vi "AWG Set Gain & Offset.vi"(6 "Pins":string[](array[string]), 8 "error in":errorcluster, 9 "Offset":dbl=0.5, 10 "Gain":dbl=0.5, 11 "Semiconductor Module Context In":T1) -> (0 "error out":errorcluster, 2 "Instruments Handle Out":refnum<k15>[](array[refnum]), 3 "Semiconductor Module Context Out":T1)   [LabVIEW 2013]
uses:
  <vilib>/NI_TestStand_SemiconductorModule/NI_TestStand_Semiconductor_Module.lvlibp/PinMap/General/SemiconductorModuleContext.ctl
  <vilib>/NI_TestStand_SemiconductorModule/NI_TestStand_Semiconductor_Module.lvlibp
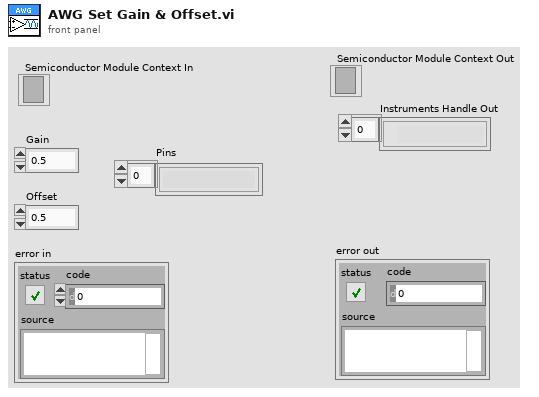
[diagram p1: front panel]
types:
  T1 = typedef "NI_TestStand_Semiconductor_Module.lvlibp/SemiconductorModuleContext.ctl" = refnum<k7>
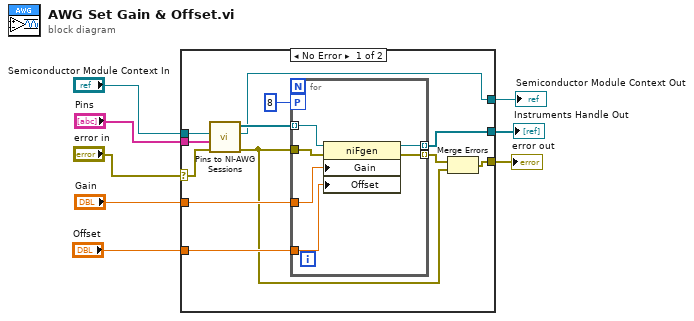
[diagram p0: block diagram]
diagram:
  n1 = case shown="No Error" "error in" {
    selector: "error in" -> [w11 w27]
    tunnel: [w20 _] -> w8
    tunnel: "Offset" -> [w19 _]
    tunnel: "Gain" -> [w18 _]
    tunnel: "Semiconductor Module Context In" -> [w17 _]
    tunnel: "Pins" -> [w16 _]
    tunnel: [w14 w27] -> w3
    tunnel: [w12 _] -> w2
    frame No Error {
      n2 = call "Pins to NI-AWG Sessions.vi"("error in (no error)"=w11, "Pins"=w16, "Semiconductor Module Context"=w17) -> ("error out"=w9:errorcluster, "Semiconductor Module Context Out"=w12:T1, "Instrument Sessions"=w15:refnum<k15>[])  [unwired: 5 in, 1 out]
      n3 = for {
        tunnel: [w26] -> w13 mode=indexing
        tunnel: [w25] -> w20 mode=indexing
        tunnel: w19 -> [w24]
        tunnel: w18 -> [w23]
        tunnel: w9 -> [w22]
        tunnel: w15 -> [w21] mode=indexing
        workers-P: 8 -> [_]
        n4 = property class="niFgen"(reference=w21, error in=w22, "Gain"=w23, "Offset"=w24) -> (reference out=w25:refnum<k15>, error out=w26:errorcluster)
      }
      n5 = Merge Errors(w13, w9) -> (w14:errorcluster)
    }
    frame Error {
    }
  }
  "error out" <- w3
  "Instruments Handle Out" <- w8
  "Semiconductor Module Context Out" <- w2
